vi "voltage.vi"(9 "u":dbl=1.0 format="%#_13g", 11 "Qube":refnum<class "Qube.lvclass">) -> (3 "Qube":refnum<class "Qube.lvclass">)   [LabVIEW 2020, in "Qube.lvclass"]
uses:
  Qube.lvclass
  Qube.lvclass/Qube.ctl
  <vilib>/Quanser/Rapid Control Prototyping Toolkit/hardware/HIL Board/_TypeSpecific/HIL Write Analog (Scalar).vi
  <vilib>/Quanser/Rapid Control Prototyping Toolkit/hardware/HIL Board/HIL Board.lvclass
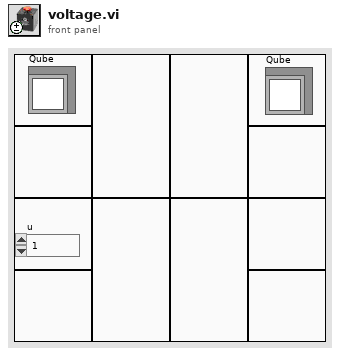
[diagram p1: front panel]
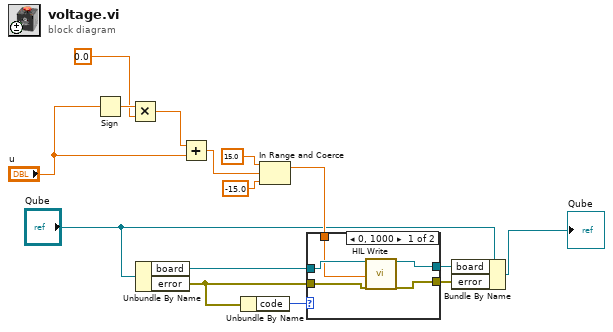
[diagram p0: block diagram]
diagram:
  n1 = Sign(1:"u") -> (0:w7:dbl)
  n2 = Multiply(x=w7, y=0.0) -> (x*y=w6:dbl)
  n3 = Unbundle By Name("Qube") -> ("board"=w15:refnum<class "HIL Board.lvclass">, "error"=w2:errorcluster)
  n4 = Add(x=w6, y="u") -> (x+y=w4:dbl)
  n5 = Unbundle By Name(w2) -> ("code"=w3:i32)
  n6 = In Range and Coerce(upper limit=15.0, x=w4, lower limit=-15.0) -> (coerced(x)=w10:dbl)  [unwired: 1 out]
  n7 = case shown="0, 1000" w3 {
    tunnel: w15 -> [w20 w22]
    tunnel: [w19 w22] -> w14
    tunnel: [w18 w21] -> w13
    tunnel: w10 -> [w17 _]
    tunnel: w2 -> [w16 w21]
    frame 0, 1000 {
      n8 = call-poly <vilib>:"HIL Write.vi"("board in"=w20, "voltage"=w17, "error in (no error)"=w16) -> ("board out"=w19:refnum<class "HIL Board.lvclass">, "error out"=w18:errorcluster)  [unwired: 15 in]
    }
    frame Default {
    }
  }
  n9 = Bundle By Name(cluster="Qube", "board"=w14, "error"=w13) -> (→"Qube":refnum<class "Qube.lvclass">)
